vi "CheckContextID.vi"(11 "context_id":string) -> (3 "valid":bool)   [LabVIEW 2013]
doc: "Every Web service method has the context_id as a parameter. This VI is just a dummy and not necessarily needed, if there is just one context available. However, in more complex situations it can be enhanced with a context-id check and a enumeration at the output for the different contexts (preferably a type definition)."
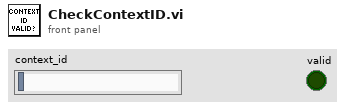
[diagram p1: front panel]
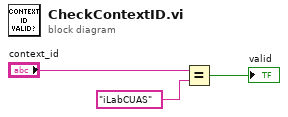
[diagram p0: block diagram]
diagram:
  n1 = Equal?(x="context_id", y="iLabCUAS") -> (x = y?=→"valid":bool)
